vi "Keithley1c_2306_Measure.vi"(11 "YTESTER测试数据":T1) -> (3 "YTESTER结论":T2)   [LabVIEW 2017]
doc: "VIDescription="
uses:
  YtCommon.lvlibp/yt`Step StepBaseInput.ctl
  YtCommon.lvlibp/yt`Step StepResult.ctl
  YtCommon.lvlibp/yt`Step TestData.ctl
  YtCommon.lvlibp/yt`Step System Queue.ctl
  Step`s VIs/YYLLGeneric/variable_W.ctl
  YtCommon.lvlibp/yt`Data-Ytester Type Data.ctl
  9150de1b-0d61-4f50-a2d9-e951e3cd4c84.vi
  72809a81-3210-4b0c-bdb6-030d0c0b3372.vi
  <vilib>/Analysis/baseanly.llb/Mean (DBL).vi
  19c99330-e7c4-4d8c-a522-00652d01c55d.vi
  c0565ce8-7c5d-4f1e-8a1f-5b5f61a1f71e.vi
  YtCommon.lvlibp
  <vilib>/Analysis/NI_AALBase.lvlib
panel:
  out "测量CH2电流mA":dbl format="%#_12f"
  out "测量CH2电压V":dbl format="%#_12f"
  out "测量CH1电流mA":dbl format="%#_12f"
  out "测量CH1电压V":dbl format="%#_12f"
  in  "YTESTER开放参数":T4={"YTESTER_BaseInput"={"isTest"=FALSE, "isSkip"=FALSE, "StepName"="Keithley2306测量", "OnPass"=enum."Next", "OnFail"=enum."Next", "ReTestNumber"=0.0}, "VISA resource"="", "测试方式"=enum."测量N次取平均（CH1+CH2）", "N次数"=1, "测量超时（s）"=10.0, "CH1电压补偿（V）"=0.0, "CH1电流补偿（mA）"=0.0, "CH2电压补偿（V）"=0.0, "CH2电流补偿（mA）"=0.0, "测电流取绝对值？"=FALSE, "CH1电压阈值上限（V）"=5.0, "CH1电压阈值下限（V）"=0.0, "CH1电流阈值上限（mA）"=50.0, "CH1电流阈值下限（mA）"=1.0, "CH2电压阈值上限（V）"=5.0, "CH2电压阈值下限（V）"=0.0, "CH2电流阈值上限（mA）"=50.0, "CH2电流阈值下限（mA）"=1.0, "测量CH1电压到变量(自定义建议#开头)"="不到变量", "测量CH1电流到变量(自定义建议#开头)"="不到变量", "测量CH2电压到变量(自定义建议#开头)"="不到变量", "测量CH2电流到变量(自定义建议#开头)"="不到变量"}
  # "2306"
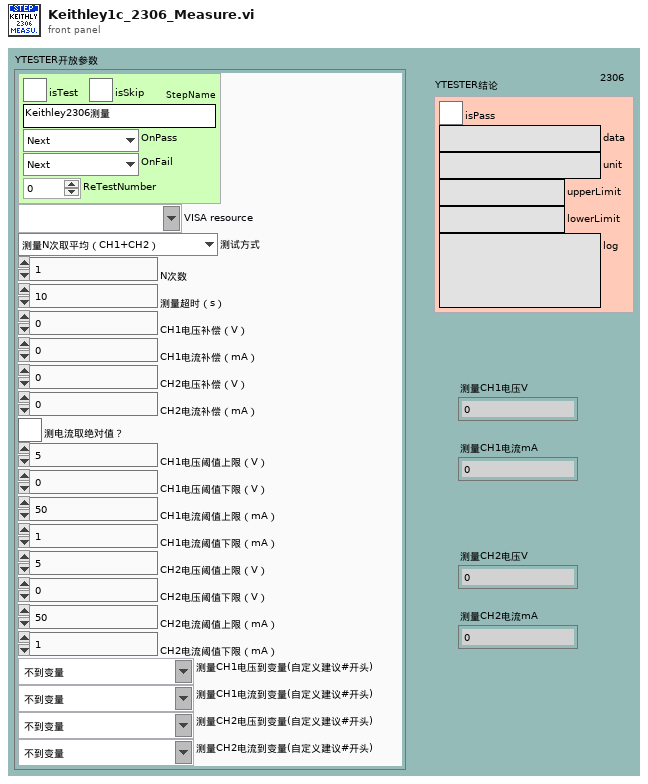
[diagram p1: front panel]
types:
  T1 = typedef "YtCommon.lvlibp/yt`Step TestData.ctl" = cluster{"Socket(From1)":i32, "SN":refnum<notifier>, "StopFlagRef":refnum<notifier>, "YT System Queue":refnum<queue>}
  T2 = typedef "YtCommon.lvlibp/yt`Step StepResult.ctl" = cluster{"isPass":bool, "data":string, "unit":string, "upperLimit":string, "lowerLimit":string, "log":string}
  T3 = typedef "YtCommon.lvlibp/yt`Step StepBaseInput.ctl" = cluster{"isTest":bool, "isSkip":bool, "StepName":string, "OnPass":enum16{"Next", "ToOVER", "Terminate"}, "OnFail":enum16{"Next", "ToOVER", "Terminate"}, "ReTestNumber":dbl}
  T4 = cluster{"YTESTER_BaseInput":T3, "VISA resource":refnum<visa-resource-name>, "测试方式":enum16{"测量N次取平均（CH1）", "测量N次取平均（CH2）", "测量N次取平均（CH1+CH2）", "满足N次阈值取平均（CH1）", "满足N次阈值取平均（CH2）", "满足N次阈值取平均（CH1+CH2）"}, "N次数":u8, "测量超时（s）":dbl, "CH1电压补偿（V）":dbl, "CH1电流补偿（mA）":dbl, "CH2电压补偿（V）":dbl, "CH2电流补偿（mA）":dbl, "测电流取绝对值？":bool, "CH1电压阈值上限（V）":dbl, "CH1电压阈值下限（V）":dbl, "CH1电流阈值上限（mA）":dbl, "CH1电流阈值下限（mA）":dbl, "CH2电压阈值上限（V）":dbl, "CH2电压阈值下限（V）":dbl, "CH2电流阈值上限（mA）":dbl, "CH2电流阈值下限（mA）":dbl, "测量CH1电压到变量(自定义建议#开头)":string, "测量CH1电流到变量(自定义建议#开头)":string, "测量CH2电压到变量(自定义建议#开头)":string, "测量CH2电流到变量(自定义建议#开头)":string}
  T5 = enum16{"测量N次取平均（CH1）", "测量N次取平均（CH2）", "测量N次取平均（CH1+CH2）", "满足N次阈值取平均（CH1）", "满足N次阈值取平均（CH2）", "满足N次阈值取平均（CH1+CH2）"}
  T6 = typedef "variable_W.ctl" = cluster{"YT_TYPE":T7, "TypeData":string[], "Tips":string}
  T7 = typedef "YtCommon.lvlibp/yt`Data-Ytester Type Data.ctl" = enum16{"NULL", "NUM", "BOOL", "TXT", "ENUM", "TIME", "PATH", "VISA", "COMBO", "ColorBox", "RadioBtn", "Array_NUM", "Array_BOOL", "Array_TXT", "Array_ENUM", "Array_PATH", "Array_COMBO"}
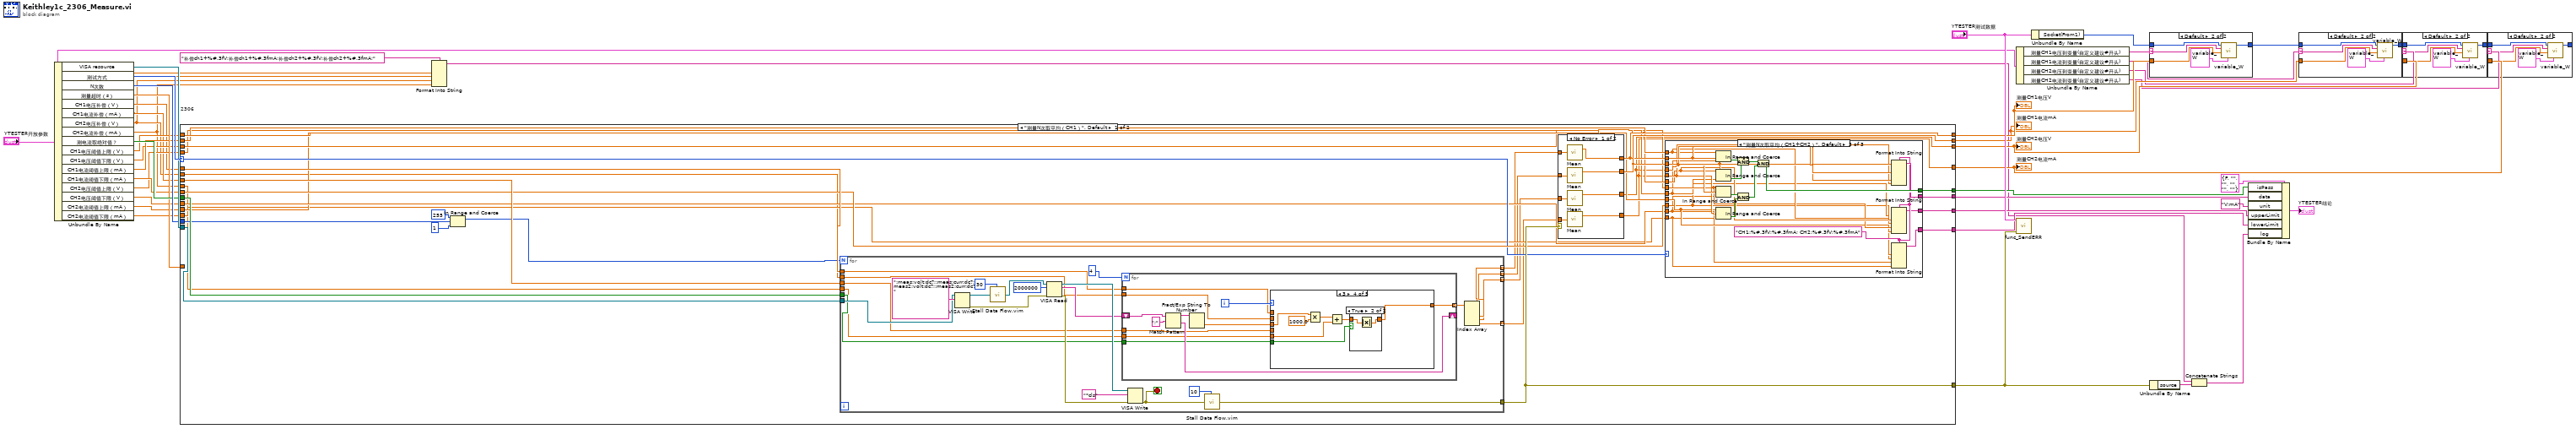
[diagram p0: block diagram]
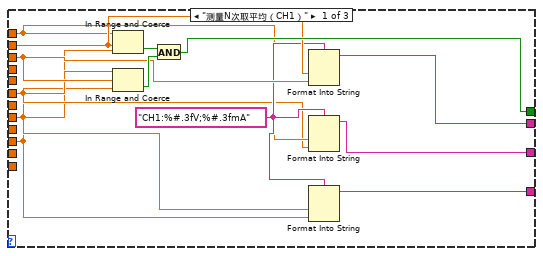
[diagram p6: hidden frame]
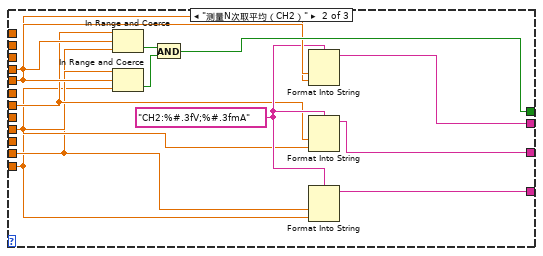
[diagram p7: hidden frame]
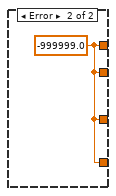
[diagram p8: hidden frame]
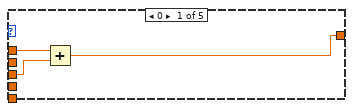
[diagram p9: hidden frame]
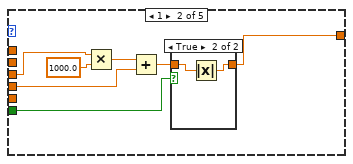
[diagram p10: hidden frame]
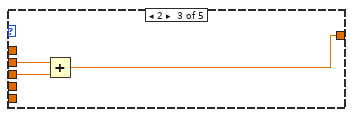
[diagram p12: hidden frame]
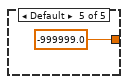
[diagram p14: hidden frame]
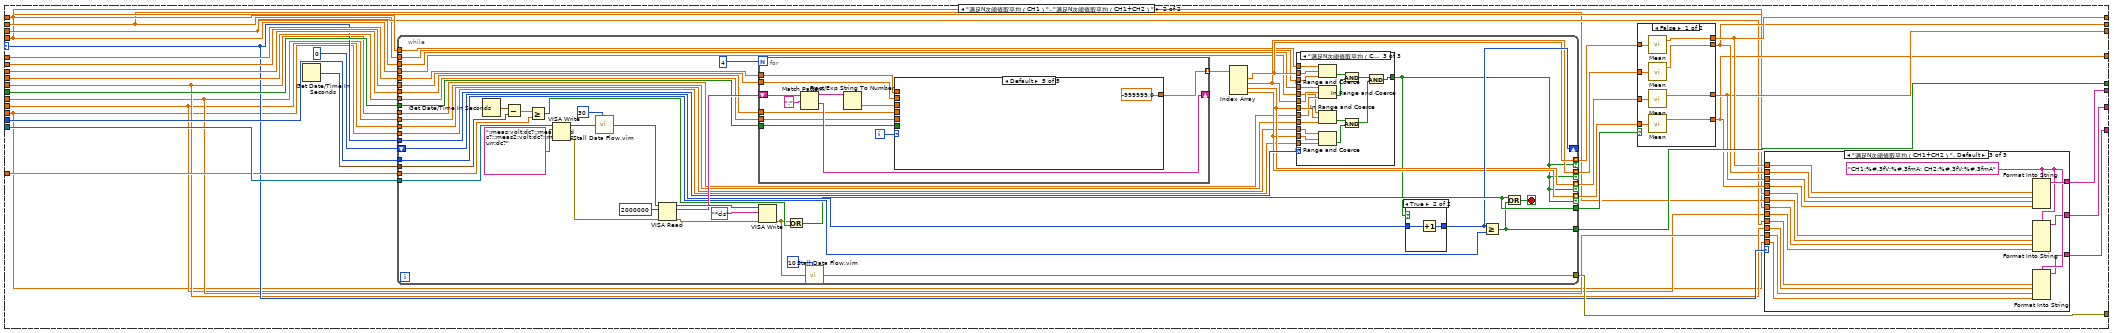
[diagram p15: hidden frame]
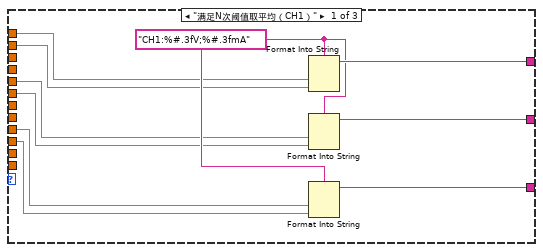
[diagram p16: hidden frame]
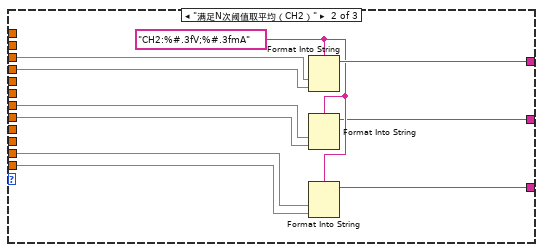
[diagram p17: hidden frame]
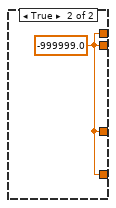
[diagram p18: hidden frame]
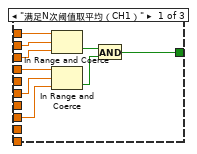
[diagram p19: hidden frame]
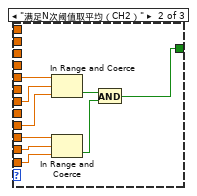
[diagram p20: hidden frame]
diagram:
  n1 = Unbundle By Name("YTESTER开放参数") -> ("VISA resource"=w41:refnum<visa-resource-name>, "测试方式"=w42:T5, "N次数"=w40:u8, "测量超时（s）"=w36:dbl, "CH1电压补偿（V）"=w7:dbl, "CH1电流补偿（mA）"=w6:dbl, "CH2电压补偿（V）"=w5:dbl, "CH2电流补偿（mA）"=w4:dbl, "测电流取绝对值？"=w39:bool, "CH1电压阈值上限（V）"=w29:dbl, "CH1电压阈值下限（V）"=w27:dbl, "CH1电流阈值上限（mA）"=w28:dbl, "CH1电流阈值下限（mA）"=w26:dbl, "CH2电压阈值上限（V）"=w24:dbl, "CH2电压阈值下限（V）"=w23:dbl, "CH2电流阈值上限（mA）"=w22:dbl, "CH2电流阈值下限（mA）"=w21:dbl)
  n2 = case "2306" shown="\"测量N次取平均（CH1）\", Default" w42 {
    selector: w42 -> [w63 w213]
    tunnel: w41 -> [w75 w224]
    tunnel: w40 -> [w49 w223]
    tunnel: w39 -> [w74 w225]
    tunnel: w7 -> [w73 w227]
    tunnel: w6 -> [w72 w226]
    tunnel: [w71 w211] -> w31
    tunnel: [w70 w212] -> w32
    tunnel: w29 -> [w68 w205]
    tunnel: w27 -> [w67 w204]
    tunnel: w28 -> [w66 w203]
    tunnel: w26 -> [w65 w202]
    tunnel: w36 -> [_ w221]
    tunnel: [w69 w219] -> w25
    tunnel: [w64 w218] -> w33
    tunnel: w24 -> [w62 w201]
    tunnel: w23 -> [w61 w200]
    tunnel: w22 -> [w60 w199]
    tunnel: w21 -> [w59 w198]
    tunnel: [w58 w210] -> w18
    tunnel: [w57 w209] -> w17
    tunnel: [w56 w208] -> w11
    tunnel: [w55 w207] -> w10
    tunnel: [w54 w206] -> w9
    tunnel: w5 -> [w45 w217]
    tunnel: w4 -> [w44 w216]
    frame "测量N次取平均（CH1）", Default {
      n3 = In Range and Coerce(upper limit=u8 255, x=w49, lower limit=u8 1) -> (coerced(x)=w46:u8)  [unwired: 1 out]
      n4 = for {
        N: w46 -> [_]
        tunnel: [w147] -> w53 mode=indexing
        tunnel: [w146] -> w52 mode=indexing
        tunnel: w75 -> [w145]
        tunnel: w74 -> [w144]
        tunnel: w73 -> [w143]
        tunnel: w72 -> [w142]
        tunnel: [w138] -> w69
        tunnel: [w137] -> w51 mode=indexing
        tunnel: [w136] -> w50 mode=indexing
        tunnel: w45 -> [w135]
        tunnel: w44 -> [w134]
        stop <- w139 stop-if-true
        n5 = VISA Write(VISA resource name=w145, write buffer=":meas:volt:dc?;:meas:curr:dc?;:meas2:volt:dc?;:meas2:curr:dc?") -> (VISA resource name out=w156:refnum<visa-resource-name>, error out=w154:errorcluster)  [unwired: 1 in, 1 out]
        n6 = call "Stall Data Flow.vim"("value in"=w156, "milliseconds to wait"=u32 30) -> ("value out"=w153:refnum<visa-resource-name>)  [unwired: 1 out]
        n7 = VISA Read(VISA resource name=w153, byte count=u32 2000000, error in (no error)=w154) -> (VISA resource name out=w157:refnum<visa-resource-name>, read buffer=w155:string, error out=w158:errorcluster)  [unwired: 1 out]
        n8 = for {
          N: 4 -> [_]
          shift-right: [w169] -> _
          shift-left: w155 -> [w170]
          tunnel: w144 -> [w164]
          tunnel: w143 -> [w163]
          tunnel: w142 -> [w162]
          tunnel: [w161] -> w141 mode=indexing
          tunnel: w135 -> [w160]
          tunnel: w134 -> [w159]
          i -> [w165]
          n9 = Match Pattern(string=w170, regular expression=";") -> (before substring=w167:string, after substring=w169:string)  [unwired: 1 in, 2 out]
          n10 = Fract/Exp String To Number(string=w167) -> (number=w166:dbl)  [unwired: 3 in, 1 out]
          n11 = case shown="3" w165 {
            tunnel: w166 -> [w173 w180 w186 w193 _]
            tunnel: [w172 w177 w185 w190 -999999.0] -> w161
            tunnel: w164 -> [_ w178 _ w191 _]
            tunnel: w163 -> [w171 _ _ _ _]
            tunnel: w162 -> [_ w174 _ _ _]
            tunnel: w160 -> [_ _ w184 _ _]
            tunnel: w159 -> [_ _ _ w187 _]
            frame 0 {
              n12 = Add(x=w171, y=w173) -> (x+y=w172:dbl)
            }
            frame 1 {
              n13 = Multiply(x=w180, y=1000.0) -> (x*y=w176:dbl)
              n14 = Add(x=w176, y=w174) -> (x+y=w175:dbl)
              n15 = case shown="True" w178 {
                tunnel: [w181 w182] -> w177
                tunnel: w175 -> [w181 w183]
                frame False {
                }
                frame True {
                  n16 = Absolute Value(x=w183) -> (abs(x)=w182:dbl)
                }
              }
            }
            frame 2 {
              n17 = Add(x=w184, y=w186) -> (x+y=w185:dbl)
            }
            frame 3 {
              n18 = Multiply(x=w193, y=1000.0) -> (x*y=w189:dbl)
              n19 = Add(x=w189, y=w187) -> (x+y=w188:dbl)
              n20 = case shown="True" w191 {
                tunnel: [w194 w195] -> w190
                tunnel: w188 -> [w194 w196]
                frame False {
                }
                frame True {
                  n21 = Absolute Value(x=w196) -> (abs(x)=w195:dbl)
                }
              }
            }
            frame Default {
            }
          }
        }
        n22 = VISA Write(VISA resource name=w157, write buffer="*cls", error in (no error)=w158) -> (error out=w139:errorcluster)  [unwired: 2 out]
        n23 = call "Stall Data Flow.vim"("value in"=w139, "milliseconds to wait"=u32 10) -> ("value out"=w138:errorcluster)  [unwired: 1 out]
        n24 = Index Array(array=w141) -> (element #1=w147:dbl, element #2=w146:dbl, element #3=w137:dbl, element #4=w136:dbl)  [unwired: 4 in]
      }
      n25 = case shown="No Error" w69 {
        tunnel: w53 -> [w132 _]
        tunnel: w52 -> [w131 _]
        tunnel: [w130 w133] -> w70
        tunnel: [w129 w133] -> w71
        tunnel: w51 -> [w128 _]
        tunnel: w50 -> [w127 _]
        tunnel: [w126 w133] -> w58
        tunnel: [w125 w133] -> w57
        frame No Error {
          n26 = call-poly <vilib>:"Mean.vi"("X"=w132) -> ("mean"=w130:dbl)  [unwired: 1 out]
          n27 = call-poly <vilib>:"Mean.vi"("X"=w131) -> ("mean"=w129:dbl)  [unwired: 1 out]
          n28 = call-poly <vilib>:"Mean.vi"("X"=w128) -> ("mean"=w126:dbl)  [unwired: 1 out]
          n29 = call-poly <vilib>:"Mean.vi"("X"=w127) -> ("mean"=w125:dbl)  [unwired: 1 out]
        }
        frame Error {
          w133 = -999999.0 ("mean")
        }
      }
      n30 = case shown="\"测量N次取平均（CH1+CH2）\", Default" w63 {
        tunnel: w70 -> [w84 _ w116]
        tunnel: w71 -> [w83 _ w115]
        tunnel: w68 -> [w79 _ w109]
        tunnel: w67 -> [w77 _ w105]
        tunnel: w66 -> [w78 _ w108]
        tunnel: w65 -> [w76 _ w104]
        tunnel: [w86 w99 w118] -> w64
        tunnel: w58 -> [_ w97 w114]
        tunnel: w57 -> [_ w96 w113]
        tunnel: w62 -> [_ w92 w107]
        tunnel: w61 -> [_ w90 w103]
        tunnel: w60 -> [_ w91 w106]
        tunnel: w59 -> [_ w89 w102]
        tunnel: [w85 w98 w117] -> w56
        tunnel: [w81 w94 w111] -> w55
        tunnel: [w80 w93 w110] -> w54
        frame "测量N次取平均（CH1）" {
          w82 = "CH1:%#.3fV;%#.3fmA" ("format string")
          n31 = In Range and Coerce(upper limit=w79, x=w84, lower limit=w77) -> (In Range?=w87:bool)  [unwired: 1 out]
          n32 = In Range and Coerce(upper limit=w78, x=w83, lower limit=w76) -> (In Range?=w88:bool)  [unwired: 1 out]
          n33 = And(x=w87, y=w88) -> (x .and. y?=w86:bool)
          n34 = Format Into String(format string=w82, w84, w83) -> (resulting string=w85:string)  [unwired: 2 in, 1 out]
          n35 = Format Into String(format string=w82, w79, w78) -> (resulting string=w81:string)  [unwired: 2 in, 1 out]
          n36 = Format Into String(format string=w82, w77, w76) -> (resulting string=w80:string)  [unwired: 2 in, 1 out]
        }
        frame "测量N次取平均（CH2）" {
          w95 = "CH2:%#.3fV;%#.3fmA" ("format string")
          n37 = In Range and Coerce(upper limit=w92, x=w97, lower limit=w90) -> (In Range?=w100:bool)  [unwired: 1 out]
          n38 = In Range and Coerce(upper limit=w91, x=w96, lower limit=w89) -> (In Range?=w101:bool)  [unwired: 1 out]
          n39 = And(x=w100, y=w101) -> (x .and. y?=w99:bool)
          n40 = Format Into String(format string=w95, w97, w96) -> (resulting string=w98:string)  [unwired: 2 in, 1 out]
          n41 = Format Into String(format string=w95, w92, w91) -> (resulting string=w94:string)  [unwired: 2 in, 1 out]
          n42 = Format Into String(format string=w95, w90, w89) -> (resulting string=w93:string)  [unwired: 2 in, 1 out]
        }
        frame "测量N次取平均（CH1+CH2）", Default {
          w112 = "CH1:%#.3fV;%#.3fmA; CH2:%#.3fV;%#.3fmA" ("format string")
          n43 = In Range and Coerce(upper limit=w109, x=w116, lower limit=w105) -> (In Range?=w123:bool)  [unwired: 1 out]
          n44 = In Range and Coerce(upper limit=w108, x=w115, lower limit=w104) -> (In Range?=w124:bool)  [unwired: 1 out]
          n45 = In Range and Coerce(upper limit=w107, x=w114, lower limit=w103) -> (In Range?=w121:bool)  [unwired: 1 out]
          n46 = In Range and Coerce(upper limit=w106, x=w113, lower limit=w102) -> (In Range?=w122:bool)  [unwired: 1 out]
          n47 = And(x=w123, y=w124) -> (x .and. y?=w120:bool)
          n48 = And(x=w121, y=w122) -> (x .and. y?=w119:bool)
          n49 = And(x=w120, y=w119) -> (x .and. y?=w118:bool)
          n50 = Format Into String(format string=w112, w116, w115, w114, w113) -> (resulting string=w117:string)  [unwired: 2 in, 1 out]
          n51 = Format Into String(format string=w112, w109, w108, w107, w106) -> (resulting string=w111:string)  [unwired: 2 in, 1 out]
          n52 = Format Into String(format string=w112, w105, w104, w103, w102) -> (resulting string=w110:string)  [unwired: 2 in, 1 out]
        }
      }
    }
    frame "满足N次阈值取平均（CH1）".."满足N次阈值取平均（CH1+CH2）" {
      n53 = Get Date/Time In Seconds() -> (seconds since 1Jan1904=w222:timestamp)
      n54 = while {
        tunnel: [w288] -> w230 mode=indexing if=w280
        tunnel: [w287] -> w229 mode=indexing if=w280
        tunnel: w224 -> [w310]
        tunnel: w225 -> [w309]
        tunnel: w227 -> [w308]
        tunnel: w226 -> [w307]
        tunnel: w205 -> [w284]
        tunnel: w204 -> [w282]
        tunnel: w203 -> [w283]
        tunnel: w202 -> [w281]
        shift-right: [w296] -> _
        shift-left: u8 0 -> [w305]
        tunnel: w223 -> [w304]
        tunnel: w222 -> [w302]
        tunnel: w221 -> [w299]
        tunnel: [w297] -> w220
        tunnel: [w293] -> w219
        tunnel: [w295] -> w218
        tunnel: w217 -> [w291]
        tunnel: w216 -> [w290]
        tunnel: w213 -> [w289]
        tunnel: [w286] -> w215 mode=indexing if=w280
        tunnel: [w285] -> w214 mode=indexing if=w280
        tunnel: w201 -> [w279]
        tunnel: w200 -> [w278]
        tunnel: w199 -> [w277]
        tunnel: w198 -> [w276]
        stop <- w301 stop-if-true
        n55 = Get Date/Time In Seconds() -> (seconds since 1Jan1904=w303:timestamp)
        n56 = Subtract(x=w303, y=w302) -> (x-y=w300:dbl)
        n57 = Greater Or Equal?(x=w300, y=w299) -> (x >= y?=w298:bool)
        n58 = VISA Write(VISA resource name=w310, write buffer=":meas:volt:dc?;:meas:curr:dc?;:meas2:volt:dc?;:meas2:curr:dc?") -> (VISA resource name out=w319:refnum<visa-resource-name>, error out=w317:errorcluster)  [unwired: 1 in, 1 out]
        n59 = call "Stall Data Flow.vim"("value in"=w319, "milliseconds to wait"=u32 30) -> ("value out"=w316:refnum<visa-resource-name>)  [unwired: 1 out]
        n60 = VISA Read(VISA resource name=w316, byte count=u32 2000000, error in (no error)=w317) -> (VISA resource name out=w320:refnum<visa-resource-name>, read buffer=w318:string, error out=w321:errorcluster)  [unwired: 1 out]
        n61 = for {
          N: 4 -> [_]
          shift-right: [w372] -> _
          shift-left: w318 -> [w373]
          tunnel: w309 -> [w367]
          tunnel: w308 -> [w366]
          tunnel: w307 -> [w365]
          tunnel: [w364] -> w306 mode=indexing
          tunnel: w291 -> [w363]
          tunnel: w290 -> [w362]
          i -> [w368]
          n62 = Match Pattern(string=w373, regular expression=";") -> (before substring=w370:string, after substring=w372:string)  [unwired: 1 in, 2 out]
          n63 = Fract/Exp String To Number(string=w370) -> (number=w369:dbl)  [unwired: 3 in, 1 out]
          n64 = case shown="Default" w368 {
            tunnel: w369 -> [w376 w379 w386 w396 _]
            tunnel: [w375 w378 w383 w393 -999999.0] -> w364
            tunnel: w367 -> [_ _ w384 w394 _]
            tunnel: w366 -> [w374 _ _ _ _]
            tunnel: w365 -> [_ _ w380 _ _]
            tunnel: w363 -> [_ w377 _ _ _]
            tunnel: w362 -> [_ _ _ w390 _]
            frame 0 {
              n65 = Add(x=w374, y=w376) -> (x+y=w375:dbl)
            }
            frame 2 {
              n66 = Add(x=w377, y=w379) -> (x+y=w378:dbl)
            }
            frame 1 {
              n67 = Multiply(x=w386, y=1000.0) -> (x*y=w382:dbl)
              n68 = Add(x=w382, y=w380) -> (x+y=w381:dbl)
              n69 = case shown="True" w384 {
                tunnel: [w387 w388] -> w383
                tunnel: w381 -> [w387 w389]
                frame False {
                }
                frame True {
                  n70 = Absolute Value(x=w389) -> (abs(x)=w388:dbl)
                }
              }
            }
            frame 3 {
              n71 = Multiply(x=w396, y=1000.0) -> (x*y=w392:dbl)
              n72 = Add(x=w392, y=w390) -> (x+y=w391:dbl)
              n73 = case shown="True" w394 {
                tunnel: [w397 w398] -> w393
                tunnel: w391 -> [w397 w399]
                frame False {
                }
                frame True {
                  n74 = Absolute Value(x=w399) -> (abs(x)=w398:dbl)
                }
              }
            }
            frame Default {
            }
          }
        }
        n75 = VISA Write(VISA resource name=w320, write buffer="*cls", error in (no error)=w321) -> (error out=w294:errorcluster)  [unwired: 2 out]
        n76 = Or(x=w294, y=w298) -> (x .or. y?=w297:bool)
        n77 = call "Stall Data Flow.vim"("value in"=w294, "milliseconds to wait"=u32 10) -> ("value out"=w293:errorcluster)  [unwired: 1 out]
        n78 = Index Array(array=w306) -> (element #1=w288:dbl, element #2=w287:dbl, element #3=w286:dbl, element #4=w285:dbl)  [unwired: 4 in]
        n79 = case shown="\"满足N次阈值取平均（CH1+CH2）\", Default" w289 {
          tunnel: [w328 w337 w352] -> w280
          tunnel: w288 -> [w327 _ w351]
          tunnel: w287 -> [w326 _ w350]
          tunnel: w286 -> [_ w336 w349]
          tunnel: w285 -> [_ w335 w348]
          tunnel: w284 -> [w325 _ w347]
          tunnel: w283 -> [w324 _ w346]
          tunnel: w282 -> [w323 _ w345]
          tunnel: w281 -> [w322 _ w344]
          tunnel: w279 -> [_ w334 w343]
          tunnel: w278 -> [_ w333 w342]
          tunnel: w277 -> [_ w332 w341]
          tunnel: w276 -> [_ w331 w340]
          frame "满足N次阈值取平均（CH1）" {
            n80 = In Range and Coerce(upper limit=w325, x=w327, lower limit=w324) -> (In Range?=w329:bool)  [unwired: 1 out]
            n81 = In Range and Coerce(upper limit=w323, x=w326, lower limit=w322) -> (In Range?=w330:bool)  [unwired: 1 out]
            n82 = And(x=w329, y=w330) -> (x .and. y?=w328:bool)
          }
          frame "满足N次阈值取平均（CH2）" {
            n83 = In Range and Coerce(upper limit=w334, x=w336, lower limit=w333) -> (In Range?=w338:bool)  [unwired: 1 out]
            n84 = In Range and Coerce(upper limit=w332, x=w335, lower limit=w331) -> (In Range?=w339:bool)  [unwired: 1 out]
            n85 = And(x=w338, y=w339) -> (x .and. y?=w337:bool)
          }
          frame "满足N次阈值取平均（CH1+CH2）", Default {
            n86 = In Range and Coerce(upper limit=w347, x=w351, lower limit=w346) -> (In Range?=w357:bool)  [unwired: 1 out]
            n87 = In Range and Coerce(upper limit=w345, x=w350, lower limit=w344) -> (In Range?=w358:bool)  [unwired: 1 out]
            n88 = In Range and Coerce(upper limit=w343, x=w349, lower limit=w342) -> (In Range?=w355:bool)  [unwired: 1 out]
            n89 = In Range and Coerce(upper limit=w341, x=w348, lower limit=w340) -> (In Range?=w356:bool)  [unwired: 1 out]
            n90 = And(x=w357, y=w358) -> (x .and. y?=w354:bool)
            n91 = And(x=w355, y=w356) -> (x .and. y?=w353:bool)
            n92 = And(x=w354, y=w353) -> (x .and. y?=w352:bool)
          }
        }
        n93 = case shown="True" w280 {
          tunnel: w305 -> [w359 w361]
          tunnel: [w359 w360] -> w296
          frame False {
          }
          frame True {
            n94 = Increment(x=w361) -> (x+1=w360:u8)
          }
        }
        n95 = Greater Or Equal?(x=w296, y=w304) -> (x >= y?=w295:bool)
        n96 = Or(x=w297, y=w295) -> (x .or. y?=w301:bool)
      }
      n97 = case shown="False" w220 {
        tunnel: [w274 w275] -> w212
        tunnel: [w273 w275] -> w211
        tunnel: w230 -> [w272 _]
        tunnel: w229 -> [w271 _]
        tunnel: w215 -> [w270 _]
        tunnel: w214 -> [w269 _]
        tunnel: [w268 w275] -> w210
        tunnel: [w267 w275] -> w209
        frame False {
          n98 = call-poly <vilib>:"Mean.vi"("X"=w272) -> ("mean"=w274:dbl)  [unwired: 1 out]
          n99 = call-poly <vilib>:"Mean.vi"("X"=w271) -> ("mean"=w273:dbl)  [unwired: 1 out]
          n100 = call-poly <vilib>:"Mean.vi"("X"=w270) -> ("mean"=w268:dbl)  [unwired: 1 out]
          n101 = call-poly <vilib>:"Mean.vi"("X"=w269) -> ("mean"=w267:dbl)  [unwired: 1 out]
        }
        frame True {
          w275 = -999999.0 ("mean")
        }
      }
      n102 = case shown="\"满足N次阈值取平均（CH1+CH2）\", Default" w213 {
        tunnel: [w240 w250 w266] -> w208
        tunnel: [w238 w248 w264] -> w207
        tunnel: [w237 w247 w263] -> w206
        tunnel: w212 -> [w236 _ w262]
        tunnel: w211 -> [w235 _ w261]
        tunnel: w210 -> [_ w246 w260]
        tunnel: w209 -> [_ w245 w259]
        tunnel: w205 -> [w234 _ w258]
        tunnel: w204 -> [w232 _ w257]
        tunnel: w203 -> [w233 _ w256]
        tunnel: w202 -> [w231 _ w255]
        tunnel: w201 -> [_ w244 w254]
        tunnel: w200 -> [_ w243 w253]
        tunnel: w199 -> [_ w242 w252]
        tunnel: w198 -> [_ w241 w251]
        frame "满足N次阈值取平均（CH1）" {
          w239 = "CH1:%#.3fV;%#.3fmA" ("format string")
          n103 = Format Into String(format string=w239, w236, w235) -> (resulting string=w240:string)  [unwired: 2 in, 1 out]
          n104 = Format Into String(format string=w239, w234, w233) -> (resulting string=w238:string)  [unwired: 2 in, 1 out]
          n105 = Format Into String(format string=w239, w232, w231) -> (resulting string=w237:string)  [unwired: 2 in, 1 out]
        }
        frame "满足N次阈值取平均（CH2）" {
          w249 = "CH2:%#.3fV;%#.3fmA" ("format string")
          n106 = Format Into String(format string=w249, w246, w245) -> (resulting string=w250:string)  [unwired: 2 in, 1 out]
          n107 = Format Into String(format string=w249, w244, w242) -> (resulting string=w248:string)  [unwired: 2 in, 1 out]
          n108 = Format Into String(format string=w249, w243, w241) -> (resulting string=w247:string)  [unwired: 2 in, 1 out]
        }
        frame "满足N次阈值取平均（CH1+CH2）", Default {
          w265 = "CH1:%#.3fV;%#.3fmA; CH2:%#.3fV;%#.3fmA" ("format string")
          n109 = Format Into String(format string=w265, w262, w261, w260, w259) -> (resulting string=w266:string)  [unwired: 2 in, 1 out]
          n110 = Format Into String(format string=w265, w258, w256, w254, w252) -> (resulting string=w264:string)  [unwired: 2 in, 1 out]
          n111 = Format Into String(format string=w265, w257, w255, w253, w251) -> (resulting string=w263:string)  [unwired: 2 in, 1 out]
        }
      }
    }
  }
  "测量CH1电压V" <- w32
  "测量CH1电流mA" <- w31
  "测量CH2电压V" <- w18
  "测量CH2电流mA" <- w17
  n112 = Format Into String(format string="补偿ch1+%#.3fV;补偿ch1+%#.3fmA;补偿ch2+%#.3fV;补偿ch2+%#.3fmA;", w7, w6, w5, w4) -> (resulting string=w3:string)  [unwired: 2 in, 1 out]
  n113 = Unbundle By Name("YTESTER开放参数") -> ("测量CH1电压到变量(自定义建议#开头)"=w15:string, "测量CH1电流到变量(自定义建议#开头)"=w14:string, "测量CH2电压到变量(自定义建议#开头)"=w13:string, "测量CH2电流到变量(自定义建议#开头)"=w12:string)
  n114 = call "func_SendERR.vi"("ERR (String\\Errclust)"=w25, "YTESTER测试数据 in"="YTESTER测试数据") -> ()  [unwired: 9 in, 1 out]
  n115 = Unbundle By Name("YTESTER测试数据") -> ("Socket(From1)"=w37:i32)
  n116 = case shown="Default" w15 {
    selector: w15 -> [_ w405]
    tunnel: w37 -> [w401 w406]
    tunnel: w32 -> [_ w403]
    tunnel: [w401 w402] -> w38
    frame "不到变量" {
    }
    frame Default {
      n117 = call "variable_W.vi"("附加的Information"=T6 {"YT_TYPE"=enum."NUM", "TypeData"=[], "Tips"="yt_Keithley电压测量缓存"}, "待写入池的输入控件"=w403, "待写入池变量名称"=w405, "函数池名称 in"=w406) -> ("函数池名称 out"=w402:i32)  [unwired: 5 in, 2 out]
    }
  }
  n118 = Unbundle By Name(w25) -> ("source"=w2:string)
  n119 = Concatenate Strings(w3, w2) -> (w1:string)
  n120 = Bundle By Name(cluster=T2 {"isPass"=FALSE, "data"="", "unit"="", "upperLimit"="", "lowerLimit"="", "log"=""} ("Result"), "isPass"=w33, "data"=w11, "unit"="V;mA", "upperLimit"=w10, "lowerLimit"=w9, "log"=w1) -> (→"YTESTER结论":T2)
  n121 = case shown="Default" w14 {
    selector: w14 -> [_ w411]
    tunnel: w38 -> [w407 w412]
    tunnel: w31 -> [_ w409]
    tunnel: [w407 w408] -> w20
    frame "不到变量" {
    }
    frame Default {
      n122 = call "variable_W.vi"("附加的Information"=T6 {"YT_TYPE"=enum."NUM", "TypeData"=[], "Tips"="yt_Keithley电流测量缓存"}, "待写入池的输入控件"=w409, "待写入池变量名称"=w411, "函数池名称 in"=w412) -> ("函数池名称 out"=w408:i32)  [unwired: 5 in, 2 out]
    }
  }
  n123 = case shown="Default" w13 {
    selector: w13 -> [_ w417]
    tunnel: w20 -> [w413 w418]
    tunnel: w18 -> [_ w415]
    tunnel: [w413 w414] -> w19
    frame "不到变量" {
    }
    frame Default {
      n124 = call "variable_W.vi"("附加的Information"=T6 {"YT_TYPE"=enum."NUM", "TypeData"=[], "Tips"="yt_Keithley电流测量缓存"}, "待写入池的输入控件"=w415, "待写入池变量名称"=w417, "函数池名称 in"=w418) -> ("函数池名称 out"=w414:i32)  [unwired: 5 in, 2 out]
    }
  }
  n125 = case shown="Default" w12 {
    selector: w12 -> [_ w423]
    tunnel: w19 -> [w419 w424]
    tunnel: w17 -> [_ w421]
    tunnel: [w419 w420] -> _
    frame "不到变量" {
    }
    frame Default {
      n126 = call "variable_W.vi"("附加的Information"=T6 {"YT_TYPE"=enum."NUM", "TypeData"=[], "Tips"="yt_Keithley电流测量缓存"}, "待写入池的输入控件"=w421, "待写入池变量名称"=w423, "函数池名称 in"=w424) -> ("函数池名称 out"=w420:i32)  [unwired: 5 in, 2 out]
    }
  }
